vi "Read classes.vi"(8 "error in (no error)":errorcluster, 11 "S4ICS in":refnum<class "S4ICS.lvclass">) -> (0 "error out":errorcluster, 2 "mechanism":T1, 3 "S4ICS out":refnum<class "S4ICS.lvclass">)   [LabVIEW 2018, in "S4ICS.lvclass"]
uses:
  S4ICS.lvclass
  State Machine/State Machine.lvclass
  RxTx/RxTx.lvclass
  S4ICS.lvclass/S4ICS.ctl
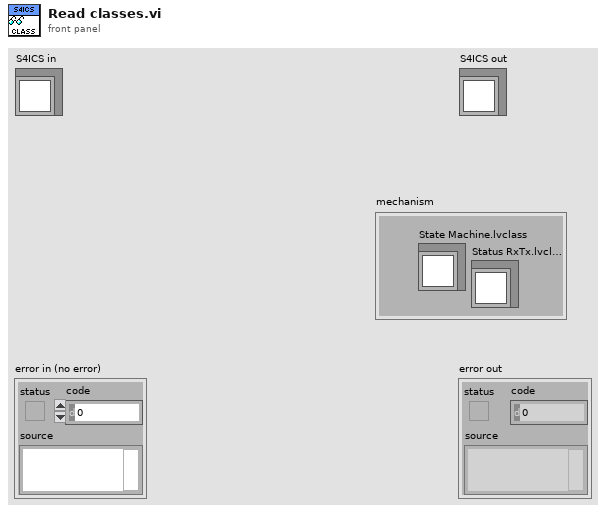
[diagram p1: front panel]
types:
  T1 = cluster{"State Machine.lvclass":refnum<class "State Machine.lvclass">, "Status RxTx.lvclass":refnum<class "RxTx.lvclass">}
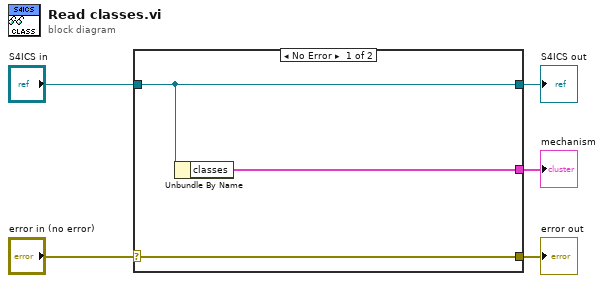
[diagram p0: block diagram]
diagram:
  n1 = case shown="No Error" "error in (no error)" {
    selector: "error in (no error)" -> [w8 w9]
    tunnel: [w8 w9] -> w4
    tunnel: [w7 w10] -> w2
    tunnel: "S4ICS in" -> [w7 w10]
    tunnel: [w6 _] -> w1
    frame No Error {
      n2 = Unbundle By Name(w7) -> ("classes"=w6:T1)
    }
    frame Error {
    }
  }
  "error out" <- w4
  "S4ICS out" <- w2
  "mechanism" <- w1
